vi "ma_SML Decimation Filter (complex input) (No State).vi"(7 "SML Decimation Filter (complex input) state":T1={"decimation settings state"={"M"=1, "stop band attenuation"=enum."84 dB", "alias protect in transition band"=TRUE, "oversampling ratio"=1.0}, "counter for garbage samples state"=0, "sml_Parameter Setting for Zoom Factor state"={"filter length * interpolation state"=0, "interpolation state"=0, "comb filter order state"=0, "CFIR par state"={"h"=[], "M"=0, "N"=0}, "LFIR par state"={"h"=[], "M"=0, "N"=0}, "CIC Stages state"=0}, "aal_CIC (complex input) state"={"aal_cascaded moving average (complex input) state"={"states"=[], "circular buffers state"=[], "circular buffer counter state"=0}, "aal_moving average with decimation by order (complex input) state"={"residue result state"=0.0+0.0i, "processed data counter state"=0}}, "sml_Cascaded Decimation Filter (complex input) CFIR state"={"unprocessed data state"=[], "final conditions state"=[], "sml_M-1 Decimator with IC (complex input) state"={"coefficients in reverse order state"=[], "max index for coefficients state"=1}}, "sml_Cascaded Decimation Filter (complex input) LFIR state"={"unprocessed data state"=[], "final conditions state"=[], "sml_M-1 Decimator with IC (complex input) state"={"coefficients in reverse order state"=[], "max index for coefficients state"=1}}} {"sml_Cascaded Decimation Filter (complex input) LFIR state"."sml_M-1 Decimator with IC (complex input) state"."coefficients in reverse order state" format="%.2f"; "sml_Cascaded Decimation Filter (complex input) CFIR state"."sml_M-1 Decimator with IC (complex input) state"."coefficients in reverse order state" format="%.2f"; "sml_Parameter Setting for Zoom Factor state"."LFIR par state"."h" format="%.2f"; "sml_Parameter Setting for Zoom Factor state"."CFIR par state"."h" format="%.2f"; "decimation settings state"."oversampling ratio" format="%.2f"; "decimation settings state"."M" min=0}, 8 "reset?":bool, 9 "truncate transition?":bool=TRUE, 10 "decimation setting":T2={"M"=1, "stop band attenuation"=enum."84 dB", "alias protect in transition band"=TRUE, "oversampling ratio"=1.0} {"oversampling ratio" format="%.2f"; "M" min=0}, 11 "x":cdb[](array[numeric]) format="%.6g") -> (0 "initial cutoff length":i32=1 min=0, 2 "y":cdb[](array[numeric]) format="%.6g", 5 "SML Decimation Filter (complex input) state":T1={"decimation settings state"={"M"=1, "stop band attenuation"=enum."84 dB", "alias protect in transition band"=TRUE, "oversampling ratio"=1.0}, "counter for garbage samples state"=0, "sml_Parameter Setting for Zoom Factor state"={"filter length * interpolation state"=0, "interpolation state"=0, "comb filter order state"=0, "CFIR par state"={"h"=[], "M"=0, "N"=0}, "LFIR par state"={"h"=[], "M"=0, "N"=0}, "CIC Stages state"=0}, "aal_CIC (complex input) state"={"aal_cascaded moving average (complex input) state"={"states"=[], "circular buffers state"=[], "circular buffer counter state"=0}, "aal_moving average with decimation by order (complex input) state"={"residue result state"=0.0+0.0i, "processed data counter state"=0}}, "sml_Cascaded Decimation Filter (complex input) CFIR state"={"unprocessed data state"=[], "final conditions state"=[], "sml_M-1 Decimator with IC (complex input) state"={"coefficients in reverse order state"=[], "max index for coefficients state"=1}}, "sml_Cascaded Decimation Filter (complex input) LFIR state"={"unprocessed data state"=[], "final conditions state"=[], "sml_M-1 Decimator with IC (complex input) state"={"coefficients in reverse order state"=[], "max index for coefficients state"=1}}} {"sml_Cascaded Decimation Filter (complex input) LFIR state"."sml_M-1 Decimator with IC (complex input) state"."coefficients in reverse order state" format="%.2f"; "sml_Cascaded Decimation Filter (complex input) CFIR state"."sml_M-1 Decimator with IC (complex input) state"."coefficients in reverse order state" format="%.2f"; "sml_Parameter Setting for Zoom Factor state"."LFIR par state"."h" format="%.2f"; "sml_Parameter Setting for Zoom Factor state"."CFIR par state"."h" format="%.2f"; "decimation settings state"."oversampling ratio" format="%.2f"; "decimation settings state"."M" min=0})   [LabVIEW 2020, in "NI_MAPro.lvlib"]
uses:
  NI_MAPro.lvlib
  NI_AALPro.lvlib
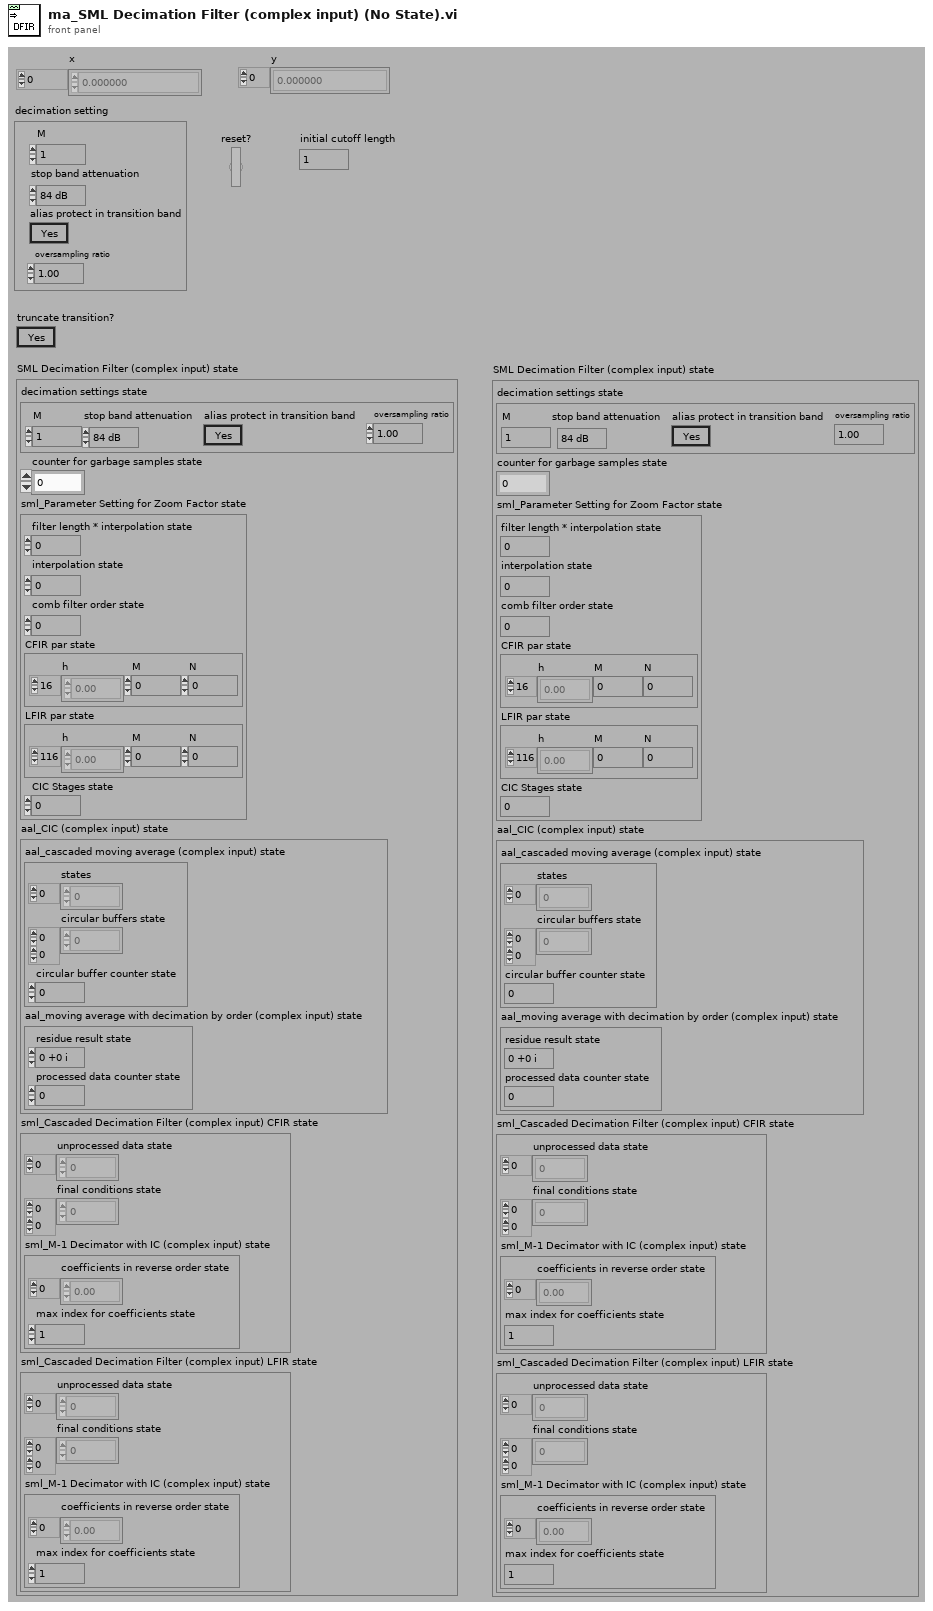
[diagram p1: front panel]
types:
  T1 = cluster{"decimation settings state":cluster{"M":i32, "stop band attenuation":enum16{"84 dB", "96 dB", "120 dB"}, "alias protect in transition band":bool, "oversampling ratio":dbl}, "counter for garbage samples state":i32, "sml_Parameter Setting for Zoom Factor state":cluster{"filter length * interpolation state":i32, "interpolation state":i32, "comb filter order state":i32, "CFIR par state":cluster{"h":dbl[], "M":i32, "N":i32}, "LFIR par state":cluster{"h":dbl[], "M":i32, "N":i32}, "CIC Stages state":i32}, "aal_CIC (complex input) state":cluster{"aal_cascaded moving average (complex input) state":cluster{"states":cdb[], "circular buffers state":cdb[][], "circular buffer counter state":i32}, "aal_moving average with decimation by order (complex input) state":cluster{"residue result state":cdb, "processed data counter state":i32}}, "sml_Cascaded Decimation Filter (complex input) CFIR state":cluster{"unprocessed data state":cdb[], "final conditions state":cdb[][], "sml_M-1 Decimator with IC (complex input) state":cluster{"coefficients in reverse order state":dbl[], "max index for coefficients state":i32}}, "sml_Cascaded Decimation Filter (complex input) LFIR state":cluster{"unprocessed data state":cdb[], "final conditions state":cdb[][], "sml_M-1 Decimator with IC (complex input) state":cluster{"coefficients in reverse order state":dbl[], "max index for coefficients state":i32}}}
  T2 = cluster{"M":i32, "stop band attenuation":enum16{"84 dB", "96 dB", "120 dB"}, "alias protect in transition band":bool, "oversampling ratio":dbl}
  T3 = cluster{"unprocessed data state":cdb[], "final conditions state":cdb[][], "sml_M-1 Decimator with IC (complex input) state":cluster{"coefficients in reverse order state":dbl[], "max index for coefficients state":i32}}
  T4 = cluster{"aal_cascaded moving average (complex input) state":cluster{"states":cdb[], "circular buffers state":cdb[][], "circular buffer counter state":i32}, "aal_moving average with decimation by order (complex input) state":cluster{"residue result state":cdb, "processed data counter state":i32}}
  T5 = cluster{"filter length * interpolation state":i32, "interpolation state":i32, "comb filter order state":i32, "CFIR par state":cluster{"h":dbl[], "M":i32, "N":i32}, "LFIR par state":cluster{"h":dbl[], "M":i32, "N":i32}, "CIC Stages state":i32}
  T6 = cluster{"M":bool, "stop band attenuation":bool, "alias protect in transition band":bool, "oversampling ratio":bool}
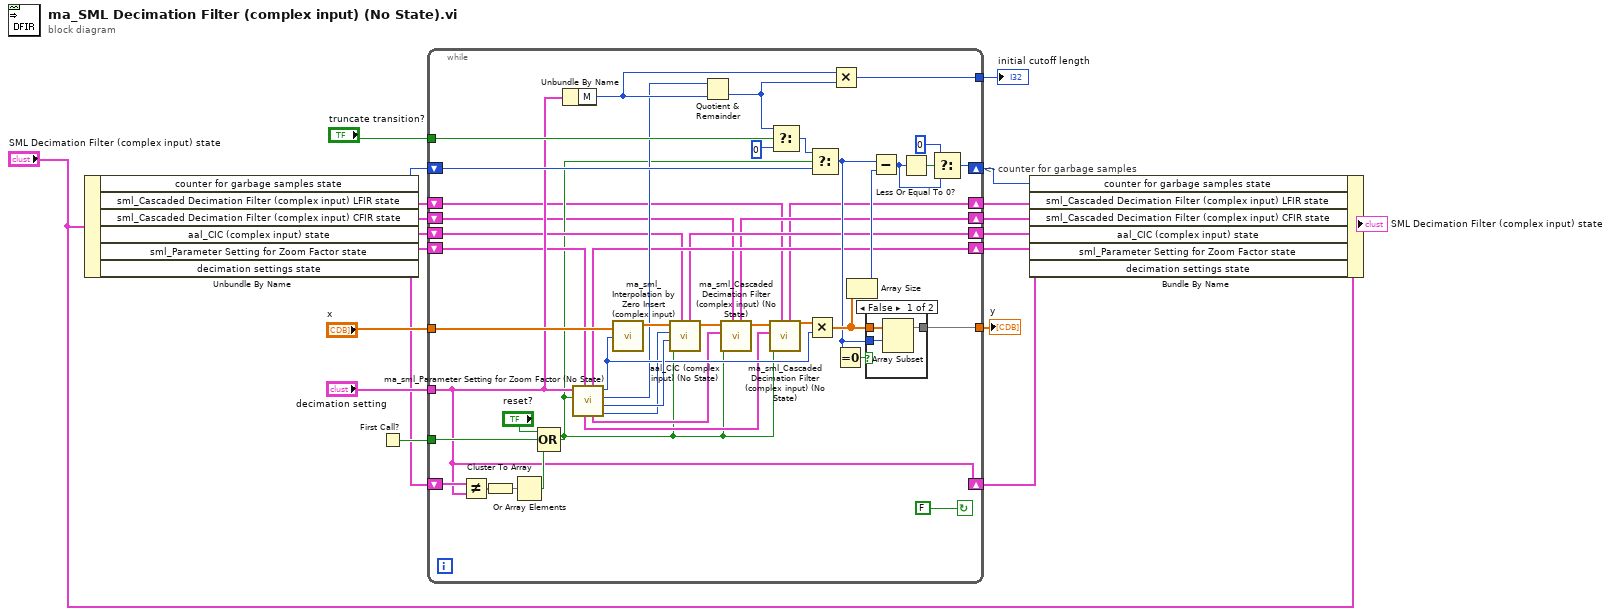
[diagram p0: block diagram]
diagram:
  # "<- counter for garbage samples"
  n1 = Unbundle By Name("SML Decimation Filter (complex input) state") -> ("counter for garbage samples state"=w9:i32, "sml_Cascaded Decimation Filter (complex input) LFIR state"=w2:T3, "sml_Cascaded Decimation Filter (complex input) CFIR state"=w6:T3, "aal_CIC (complex input) state"=w8:T4, "sml_Parameter Setting for Zoom Factor state"=w13:T5, "decimation settings state"=w14:T2)
  n2 = First Call?() -> (First Call?: T/F=w17:bool)
  n3 = while {
    tunnel: [w42] -> w15
    tunnel: "truncate transition?" -> [w43]
    tunnel: w17 -> [w44]
    tunnel: "x" -> [w49]
    tunnel: "decimation setting" -> [w39]
    shift-left: w9 -> [w58]
    shift-right: [w54] -> w4
    tunnel: [w59] -> w20
    shift-left: w14 -> [w63]
    shift-right: [w39] -> w10
    shift-right: [w23] -> w5
    shift-left: w6 -> [w24]
    shift-right: [w31] -> w7
    shift-left: w8 -> [w32]
    shift-right: [w33] -> w11
    shift-left: w13 -> [w34]
    shift-right: [w21] -> w1
    shift-left: w2 -> [w22]
    stop <- FALSE continue-if-true
    n4 = Not Equal?(x=w63, y=w39) -> (x != y?=w62:T6)
    n5 = Cluster To Array(cluster=w62) -> (array=w61:bool[])
    n6 = Or Array Elements(Boolean array=w61) -> (logical OR=w45:bool)
    n7 = Compound Arithmetic op=OR("reset?", w44, w45) -> (w26:bool)
    n8 = Unbundle By Name(w39) -> ("M"=w40:i32)
    n9 = call "ma_sml_Parameter Setting for Zoom Factor (No State).vi"("sml_Parameter Setting for Zoom Factor state in"=w34, "Reset"=w26, "zoom settings"=w39) -> ("comb filter order"=w35:i32, "CIC Stages"=w38:i32, "filter length"=w36:i32, "interpolation"=w37:i32, "CFIR par"=w30:cluster{"h":dbl[], "M":i32, "N":i32}, "sml_Parameter Setting for Zoom Factor state out"=w33:T5, "LFIR par"=w27:cluster{"h":dbl[], "M":i32, "N":i32})  [unwired: 2 out]
    n10 = call "ma_sml_Interpolation by Zero Insert (complex input).vi"("L"=w37, "x"=w49) -> ("y"=w64:cdb[])
    n11 = call "aal_CIC (complex input) (No State).vi"("aal_CIC (complex input) state in"=w32, "Reset"=w26, "Stages"=w38, "N"=w35, "x"=w64) -> ("y"=w29:cdb[], "aal_CIC (complex input) state out"=w31:T4)  [unwired: 5 out]
    n12 = Quotient & Remainder(x=w36, y=w40) -> (floor(x/y)=w41:i32)  [unwired: 1 out]
    n13 = call "ma_sml_Cascaded Decimation Filter (complex input) (No State).vi"("reset?"=w26, "sml_Cascaded Decimation Filter (complex input) state in"=w24, "filter specification"=w30, "x"=w29) -> ("y"=w28:cdb[], "sml_Cascaded Decimation Filter (complex input) state out"=w23:T3)  [unwired: 6 out]
    n14 = call "ma_sml_Cascaded Decimation Filter (complex input) (No State).vi"("reset?"=w26, "sml_Cascaded Decimation Filter (complex input) state in"=w22, "filter specification"=w27, "x"=w28) -> ("y"=w25:cdb[], "sml_Cascaded Decimation Filter (complex input) state out"=w21:T3)  [unwired: 6 out]
    n15 = Select(t=w41, s=w43, f=0) -> (s? t:f=w47:i32)
    n16 = Multiply(x=w25, y=w37) -> (x*y=w57:cdb[])
    n17 = Select(t=w47, s=w26, f=w58) -> (s? t:f=w51:i32)
    n18 = Multiply(x=w40, y=w41) -> (x*y=w42:i32)
    n19 = Equal To 0?(x=w51) -> (x = 0?=w50:bool)
    n20 = Array Size(array=w57) -> (size(s)=w56:i32)
    n21 = case shown="False" w50 {
      tunnel: [w67 w68] -> w59
      tunnel: w57 -> [w66 w68]
      tunnel: w51 -> [w65 _]
      frame False {
        n22 = Array Subset(array=w66, index=w65) -> (w67:cdb[])  [unwired: 1 in]
      }
      frame True {
      }
    }
    n23 = Subtract(x=w51, y=w56) -> (x-y=w53:i32)
    n24 = Less Or Equal To 0?(x=w53) -> (x <= 0?=w55:bool)
    n25 = Select(t=0, s=w55, f=w53) -> (s? t:f=w54:i32)
  }
  "y" <- w20
  "initial cutoff length" <- w15
  n26 = Bundle By Name(cluster="SML Decimation Filter (complex input) state", "counter for garbage samples state"=w4, "sml_Cascaded Decimation Filter (complex input) LFIR state"=w1, "sml_Cascaded Decimation Filter (complex input) CFIR state"=w5, "aal_CIC (complex input) state"=w7, "sml_Parameter Setting for Zoom Factor state"=w11, "decimation settings state"=w10) -> (→"SML Decimation Filter (complex input) state":T1)
